vi "Instantaneous Flicker Sensation.vi"(0 "voltage waveforms":waveform(dbl)[](array[waveform]), 1 "reset? (F)":bool, 5 "voltage system":enum16{"120 V", "230 V"}(ring), 7 "half-cycle voltage RMS":T1(array[cluster]), 9 "system info in":refnum<class "EP System Info.lvclass">, 11 "error in (no error)":errorcluster) -> (4 "Pinst":waveform(dbl)[](array[waveform]), 10 "system info out":refnum<class "EP System Info.lvclass">, 15 "error out":errorcluster)   [LabVIEW 2014, in "NI_EP_Power Quality.lvlib"]
doc: "Calculates the instantaneous flicker values of a voltage waveform, according to IEC 61000-4-15:2010.\n\nThis VI supports measuring single-bus single-line or multiple-bus single-line systems."
uses:
  <vilib>/addons/Electrical Power/PQ/NI_EP_Power Quality.lvlib
  <vilib>/addons/Electrical Power/PQ/Common/Classes/System Info/EP System Info.lvclass
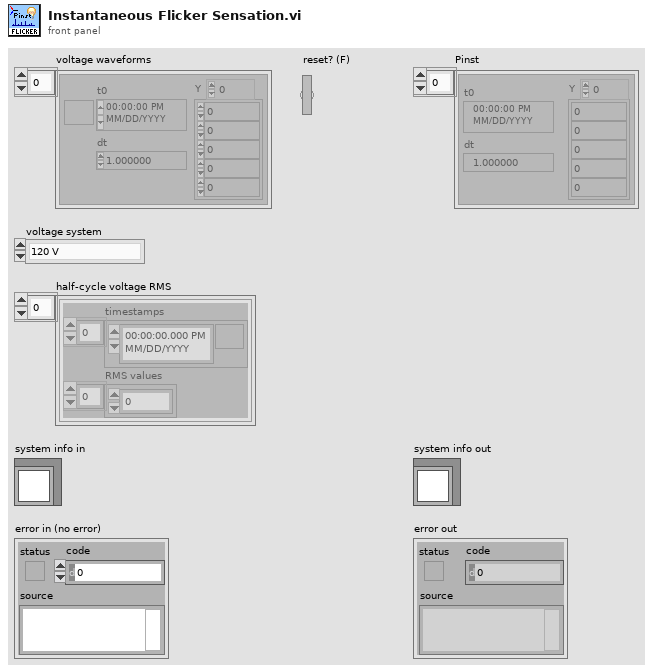
[diagram p1: front panel]
types:
  T1 = cluster{"timestamps":timestamp[], "RMS values":dbl[]}[]
  T2 = cluster{"timestamps":timestamp[], "RMS values":dbl[]}
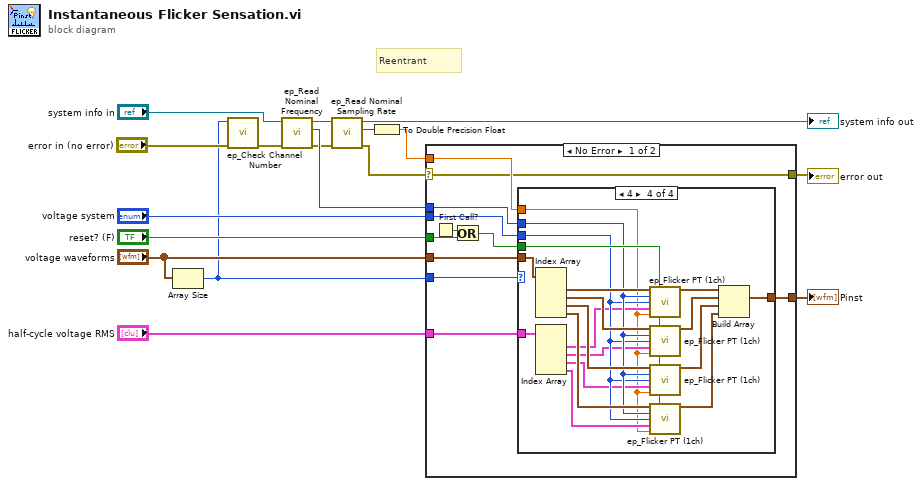
[diagram p0: block diagram]
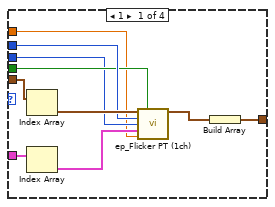
[diagram p2: hidden frame]
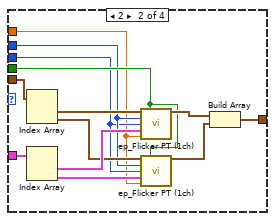
[diagram p3: hidden frame]
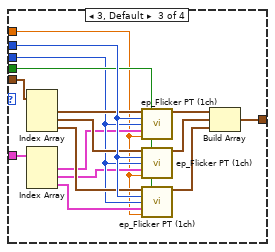
[diagram p4: hidden frame]
diagram:
  # "Reentrant"
  n1 = Array Size(array="voltage waveforms") -> (size(s)=w4:i32)
  n2 = call <vilib>:"ep_Check Channel Number.vi"("channel number"=w4, "error in (no error)"="error in (no error)") -> ("error out"=w3:errorcluster)  [unwired: 13 in]
  n3 = call <vilib>:"ep_Read Nominal Frequency.vi"("error in (no error)"=w3, "system info in"="system info in") -> ("error out"=w6:errorcluster, "nominal frequency"=w9:enum16{"50 Hz", "60 Hz"}, "system info out"=w7:refnum<class "EP System Info.lvclass">)  [unwired: 6 in, 1 out]
  n4 = call <vilib>:"ep_Read Nominal Sampling Rate.vi"("error in (no error)"=w6, "system info in"=w7) -> ("error out"=w2:errorcluster, "nominal sampling rate (Hz)"=w8:u16, "system info out"=→"system info out":refnum<class "EP System Info.lvclass">)  [unwired: 7 in]
  n5 = To Double Precision Float(number=w8) -> (double precision float=w5:dbl)
  n6 = case shown="No Error" w2 {
    selector: w2 -> [w18 w87]
    tunnel: "half-cycle voltage RMS" -> [w28 _]
    tunnel: "voltage system" -> [w27 _]
    tunnel: [w26 _] -> w14
    tunnel: "reset? (F)" -> [w25 _]
    tunnel: "voltage waveforms" -> [w24 _]
    tunnel: w9 -> [w23 _]
    tunnel: w5 -> [w22 _]
    tunnel: w4 -> [w19 _]
    tunnel: [w18 w87] -> w1
    frame No Error {
      n7 = First Call?() -> (First Call?: T/F=w21:bool)
      n8 = Or(x=w21, y=w25) -> (x .or. y?=w20:bool)
      n9 = case shown="4" w19 {
        tunnel: w24 -> [w38 w51 w67 w86]
        tunnel: w20 -> [w33 w45 w60 w78]
        tunnel: w23 -> [w34 w43 w65 w75]
        tunnel: [w37 w50 w66 w85] -> w26
        tunnel: w27 -> [w32 w42 w57 w74]
        tunnel: w28 -> [w31 w47 w56 w73]
        tunnel: w22 -> [w29 w40 w52 w68]
        frame 1 {
          n10 = Index Array(array=w38) -> (element=w36:waveform(dbl))  [unwired: 1 in]
          n11 = Index Array(array=w31) -> (element=w30:T2)  [unwired: 1 in]
          n12 = call <vilib>:"ep_Flicker PT (1ch).vi"("voltage waveform"=w36, "init"=w33, "nominal frequency"=w34, "voltage system"=w32, "RMS (1/2) (half cycle)"=w30, "nominal sampling rate [Hz]"=w29) -> ("instantaneous flicker Pinst (Output 5)"=w35:waveform(dbl))  [unwired: 9 in]
          n13 = Build Array(w35) -> (w37:waveform(dbl)[])
        }
        frame 2 {
          n14 = Index Array(array=w51) -> (element #1=w49:waveform(dbl), element #2=w44:waveform(dbl))  [unwired: 2 in]
          n15 = Index Array(array=w47) -> (element #1=w46:T2, element #2=w41:T2)  [unwired: 2 in]
          n16 = call <vilib>:"ep_Flicker PT (1ch).vi"("voltage waveform"=w49, "init"=w45, "nominal frequency"=w43, "voltage system"=w42, "RMS (1/2) (half cycle)"=w46, "nominal sampling rate [Hz]"=w40) -> ("instantaneous flicker Pinst (Output 5)"=w48:waveform(dbl))  [unwired: 9 in]
          n17 = call <vilib>:"ep_Flicker PT (1ch).vi"("voltage waveform"=w44, "init"=w45, "nominal frequency"=w43, "voltage system"=w42, "RMS (1/2) (half cycle)"=w41, "nominal sampling rate [Hz]"=w40) -> ("instantaneous flicker Pinst (Output 5)"=w39:waveform(dbl))  [unwired: 9 in]
          n18 = Build Array(w48, w39) -> (w50:waveform(dbl)[])
        }
        frame 3, Default {
          n19 = Index Array(array=w67) -> (element #1=w64:waveform(dbl), element #2=w62:waveform(dbl), element #3=w61:waveform(dbl))  [unwired: 3 in]
          n20 = Index Array(array=w56) -> (element #1=w54:T2, element #2=w55:T2, element #3=w53:T2)  [unwired: 3 in]
          n21 = call <vilib>:"ep_Flicker PT (1ch).vi"("voltage waveform"=w64, "init"=w60, "nominal frequency"=w65, "voltage system"=w57, "RMS (1/2) (half cycle)"=w54, "nominal sampling rate [Hz]"=w52) -> ("instantaneous flicker Pinst (Output 5)"=w63:waveform(dbl))  [unwired: 9 in]
          n22 = call <vilib>:"ep_Flicker PT (1ch).vi"("voltage waveform"=w62, "init"=w60, "nominal frequency"=w65, "voltage system"=w57, "RMS (1/2) (half cycle)"=w55, "nominal sampling rate [Hz]"=w52) -> ("instantaneous flicker Pinst (Output 5)"=w59:waveform(dbl))  [unwired: 9 in]
          n23 = call <vilib>:"ep_Flicker PT (1ch).vi"("voltage waveform"=w61, "init"=w60, "nominal frequency"=w65, "voltage system"=w57, "RMS (1/2) (half cycle)"=w53, "nominal sampling rate [Hz]"=w52) -> ("instantaneous flicker Pinst (Output 5)"=w58:waveform(dbl))  [unwired: 9 in]
          n24 = Build Array(w63, w59, w58) -> (w66:waveform(dbl)[])
        }
        frame 4 {
          n25 = Index Array(array=w86) -> (element #1=w84:waveform(dbl), element #2=w82:waveform(dbl), element #3=w81:waveform(dbl), element #4=w77:waveform(dbl))  [unwired: 4 in]
          n26 = Index Array(array=w73) -> (element #1=w72:T2, element #2=w71:T2, element #3=w70:T2, element #4=w69:T2)  [unwired: 4 in]
          n27 = call <vilib>:"ep_Flicker PT (1ch).vi"("voltage waveform"=w84, "init"=w78, "nominal frequency"=w75, "voltage system"=w74, "RMS (1/2) (half cycle)"=w72, "nominal sampling rate [Hz]"=w68) -> ("instantaneous flicker Pinst (Output 5)"=w83:waveform(dbl))  [unwired: 9 in]
          n28 = call <vilib>:"ep_Flicker PT (1ch).vi"("voltage waveform"=w82, "init"=w78, "nominal frequency"=w75, "voltage system"=w74, "RMS (1/2) (half cycle)"=w71, "nominal sampling rate [Hz]"=w68) -> ("instantaneous flicker Pinst (Output 5)"=w80:waveform(dbl))  [unwired: 9 in]
          n29 = call <vilib>:"ep_Flicker PT (1ch).vi"("voltage waveform"=w81, "init"=w78, "nominal frequency"=w75, "voltage system"=w74, "RMS (1/2) (half cycle)"=w70, "nominal sampling rate [Hz]"=w68) -> ("instantaneous flicker Pinst (Output 5)"=w79:waveform(dbl))  [unwired: 9 in]
          n30 = call <vilib>:"ep_Flicker PT (1ch).vi"("voltage waveform"=w77, "init"=w78, "nominal frequency"=w75, "voltage system"=w74, "RMS (1/2) (half cycle)"=w69, "nominal sampling rate [Hz]"=w68) -> ("instantaneous flicker Pinst (Output 5)"=w76:waveform(dbl))  [unwired: 9 in]
          n31 = Build Array(w83, w80, w79, w76) -> (w85:waveform(dbl)[])
        }
      }
    }
    frame Error {
    }
  }
  "error out" <- w1
  "Pinst" <- w14
